vi "Sort_Dust_Array.vi"(1 "Order by...":T1(ring), 2 "Array In":T2[](array[typedef])) -> (0 "Array out":T2[](array[typedef]))   [LabVIEW 2013]
doc: "Takes a given array of dust_type elements, and returns the same array, ordered by the given column. Ordering by \"dust_name\" will order first by \"dust_name\", second by the \"dust_type\", and third by \"batch_no\"."
uses:
  Controls/Dust_list.ctl
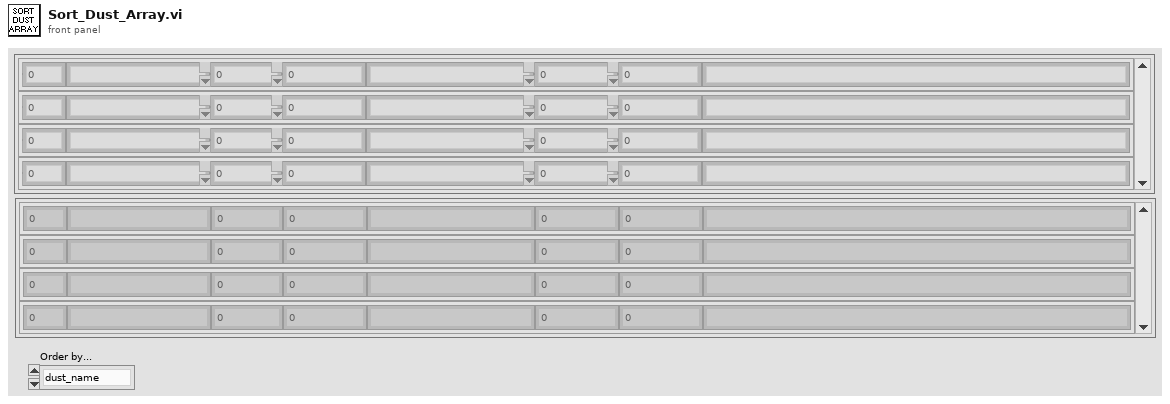
[diagram p1: front panel]
types:
  T1 = enum16{"dust_name", "dust_density", "source_weight", "bottle_weight", "dust_weight"}
  T2 = typedef "dust_list.ctl" = cluster{"id_dust_type":i32, "dust_name":string, "dust_density":dbl, "source_weight":dbl, "size":string, "bottle_weight":dbl, "dust_mass":dbl, "comments":string}
  T3 = cluster{"dust_name":string, "dust_type":i32, "batch_no":i32, "index":i32}
  T4 = cluster{"dust_name":string, "dust_type":i32, "batch_no":i32, "index":i32}[]
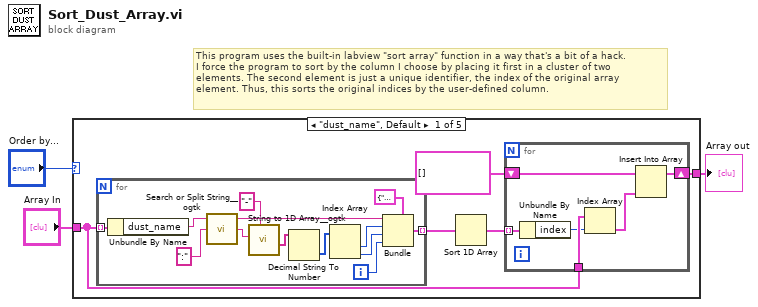
[diagram p0: block diagram]
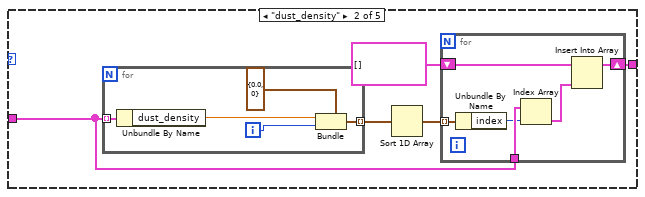
[diagram p2: hidden frame]
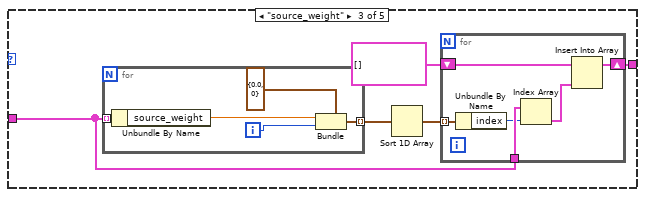
[diagram p3: hidden frame]
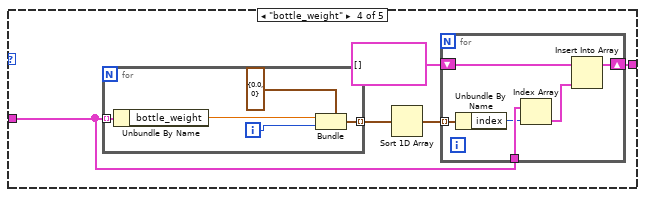
[diagram p4: hidden frame]
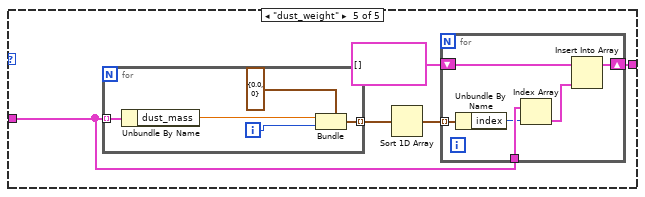
[diagram p5: hidden frame]
diagram:
  # "This program uses the built-in labview \"sort array\" function in a way that's a bit of a hack.\nI force the program to sort by the column I choose by placing it first in a cluster of two\nelements. The second element is just a unique identifier, the index of the original array\nelement. Thus, this sorts the original indices by the user-defined column."
  n1 = case shown="\"dust_name\", Default" "Order by..." {
    tunnel: "Array In" -> [w6 w30 w46 w62 w78]
    tunnel: [w4 w28 w44 w60 w76] -> w1
    frame "dust_name", Default {
      n2 = for {
        tunnel: w6 -> [w27] mode=indexing
        tunnel: [w26] -> w5 mode=indexing
        i -> [w21]
        n3 = Unbundle By Name(w27) -> ("dust_name"=w24:string)
        n4 = call <userlib>:"Search or Split String__ogtk.vi"("search string/char (-)"=":", "string"=w24) -> ("substring after match"=w20:string, "substring before match"=w22:string)  [unwired: 1 in, 1 out]
        n5 = call <userlib>:"String to 1D Array__ogtk.vi"("delimiter (Tab)"="-", "string"=w20) -> ("Array of Strings"=w18:string[])  [unwired: 9 in]
        n6 = Decimal String To Number(string=w18) -> (number=w17:i32[])  [unwired: 2 in, 1 out]
        n7 = Index Array(array=w17) -> (element #1=w16:i32, element #2=w15:i32)  [unwired: 2 in]
        n8 = Bundle(cluster=T3 {"dust_name"="", "dust_type"=0, "batch_no"=0, "index"=0}, "dust_name"=w22, "dust_type"=w16, "batch_no"=w15, "index"=w21) -> (w26:T3)
      }
      n9 = Sort 1D Array(array=w5) -> (sorted array=w8:T4)
      n10 = for {
        tunnel: w8 -> [w14] mode=indexing
        shift-right: [w12] -> w4
        shift-left: T2[] [] ("Array In") -> [w13]
        tunnel: w6 -> [w11]
        n11 = Unbundle By Name(w14) -> ("index"=w9:i32)
        n12 = Index Array(array=w11, index=w9) -> (element=w10:T2)
        n13 = Insert Into Array(array=w13, new element=w10) -> (w12:T2[])  [unwired: 1 in]
      }
    }
    frame "dust_density" {
      n14 = for {
        tunnel: w30 -> [w43] mode=indexing
        tunnel: [w41] -> w29 mode=indexing
        i -> [w40]
        n15 = Unbundle By Name(w43) -> ("dust_density"=w42:dbl)
        n16 = Bundle(cluster=cluster{"dust_name":dbl, "index":i32} {"dust_name"=0.0, "index"=0}, "dust_name"=w42, "index"=w40) -> (w41:cluster{"dust_name":dbl, "index":i32})
      }
      n17 = Sort 1D Array(array=w29) -> (sorted array=w32:cluster{"dust_name":dbl, "index":i32}[])
      n18 = for {
        tunnel: w32 -> [w38] mode=indexing
        shift-right: [w36] -> w28
        shift-left: T2[] [] ("Array In") -> [w37]
        tunnel: w30 -> [w35]
        n19 = Unbundle By Name(w38) -> ("index"=w33:i32)
        n20 = Index Array(array=w35, index=w33) -> (element=w34:T2)
        n21 = Insert Into Array(array=w37, new element=w34) -> (w36:T2[])  [unwired: 1 in]
      }
    }
    frame "source_weight" {
      n22 = for {
        tunnel: w46 -> [w59] mode=indexing
        tunnel: [w57] -> w45 mode=indexing
        i -> [w56]
        n23 = Unbundle By Name(w59) -> ("source_weight"=w58:dbl)
        n24 = Bundle(cluster=cluster{"dust_name":dbl, "index":i32} {"dust_name"=0.0, "index"=0}, "dust_name"=w58, "index"=w56) -> (w57:cluster{"dust_name":dbl, "index":i32})
      }
      n25 = Sort 1D Array(array=w45) -> (sorted array=w48:cluster{"dust_name":dbl, "index":i32}[])
      n26 = for {
        tunnel: w48 -> [w54] mode=indexing
        shift-right: [w52] -> w44
        shift-left: T2[] [] ("Array In") -> [w53]
        tunnel: w46 -> [w51]
        n27 = Unbundle By Name(w54) -> ("index"=w49:i32)
        n28 = Index Array(array=w51, index=w49) -> (element=w50:T2)
        n29 = Insert Into Array(array=w53, new element=w50) -> (w52:T2[])  [unwired: 1 in]
      }
    }
    frame "bottle_weight" {
      n30 = for {
        tunnel: w62 -> [w75] mode=indexing
        tunnel: [w73] -> w61 mode=indexing
        i -> [w72]
        n31 = Unbundle By Name(w75) -> ("bottle_weight"=w74:dbl)
        n32 = Bundle(cluster=cluster{"dust_name":dbl, "index":i32} {"dust_name"=0.0, "index"=0}, "dust_name"=w74, "index"=w72) -> (w73:cluster{"dust_name":dbl, "index":i32})
      }
      n33 = Sort 1D Array(array=w61) -> (sorted array=w64:cluster{"dust_name":dbl, "index":i32}[])
      n34 = for {
        tunnel: w64 -> [w70] mode=indexing
        shift-right: [w68] -> w60
        shift-left: T2[] [] ("Array In") -> [w69]
        tunnel: w62 -> [w67]
        n35 = Unbundle By Name(w70) -> ("index"=w65:i32)
        n36 = Index Array(array=w67, index=w65) -> (element=w66:T2)
        n37 = Insert Into Array(array=w69, new element=w66) -> (w68:T2[])  [unwired: 1 in]
      }
    }
    frame "dust_weight" {
      n38 = for {
        tunnel: w78 -> [w91] mode=indexing
        tunnel: [w89] -> w77 mode=indexing
        i -> [w88]
        n39 = Unbundle By Name(w91) -> ("dust_mass"=w90:dbl)
        n40 = Bundle(cluster=cluster{"dust_name":dbl, "index":i32} {"dust_name"=0.0, "index"=0}, "dust_name"=w90, "index"=w88) -> (w89:cluster{"dust_name":dbl, "index":i32})
      }
      n41 = Sort 1D Array(array=w77) -> (sorted array=w80:cluster{"dust_name":dbl, "index":i32}[])
      n42 = for {
        tunnel: w80 -> [w86] mode=indexing
        shift-right: [w84] -> w76
        shift-left: T2[] [] ("Array In") -> [w85]
        tunnel: w78 -> [w83]
        n43 = Unbundle By Name(w86) -> ("index"=w81:i32)
        n44 = Index Array(array=w83, index=w81) -> (element=w82:T2)
        n45 = Insert Into Array(array=w85, new element=w82) -> (w84:T2[])  [unwired: 1 in]
      }
    }
  }
  "Array out" <- w1
